vi "Initialization Check.vi"(8 "error in (no error)":errorcluster, 11 "VI in":refnum<vi>) -> (0 "error out":errorcluster)   [LabVIEW 2015]
doc: "This will check for required folder. If any folders are not found a folder will be created. This VI will also initialize all values."
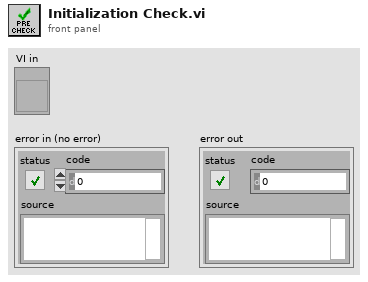
[diagram p1: front panel]
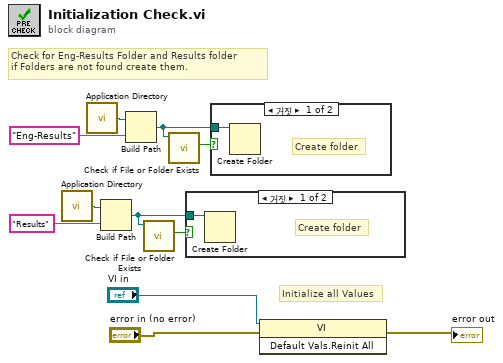
[diagram p0: block diagram]
diagram:
  # "Initialize all Values"
  # "Check for Eng-Results Folder and Results folder\nif Folders are not found create them."
  n1 = call <vilib>:"Application Directory.vi"() -> ("Application Directory"=w7:path)
  n2 = call <vilib>:"Application Directory.vi"() -> ("Application Directory"=w10:path)
  n3 = Build Path(base path=w7, name or relative path="Results") -> (appended path=w4:path)
  n4 = Build Path(base path=w10, name or relative path="Eng-Results") -> (appended path=w8:path)
  n5 = call <vilib>:"Check if File or Folder Exists.vi"("path"=w4) -> ("file or folder exists?"=w5:bool)  [unwired: 8 in, 2 out]
  n6 = call <vilib>:"Check if File or Folder Exists.vi"("path"=w8) -> ("file or folder exists?"=w11:bool)  [unwired: 8 in, 2 out]
  n7 = case shown="거짓" w5 {
    tunnel: w4 -> [w12 _]
    frame False {
      # "Create folder"
      n8 = Create Folder(path (use dialog)=w12) -> ()  [unwired: 2 in, 3 out]
    }
    frame True {
      # "Folder Exists"
    }
  }
  n9 = case shown="거짓" w11 {
    tunnel: w8 -> [w13 _]
    frame False {
      # "Create folder"
      n10 = Create Folder(path (use dialog)=w13) -> ()  [unwired: 2 in, 3 out]
    }
    frame True {
      # "Folder Exists"
    }
  }
  n11 = invoke class="VI" method="Default Vals.Reinit All"(reference="VI in", error in="error in (no error)") -> (error out=→"error out":errorcluster)  [unwired: 1 in, 2 out]
